vi "HysteresisExample.vi"() -> ()   [LabVIEW 2020]
panel:
  out "Output":dbl
  out "Waveform Chart":dbl(graph)
  out "ON":bool
  in  "High threshold":dbl=11.0
  in  "Low threshold":dbl=9.0
  in  "Start":bool
  in  "stop":bool
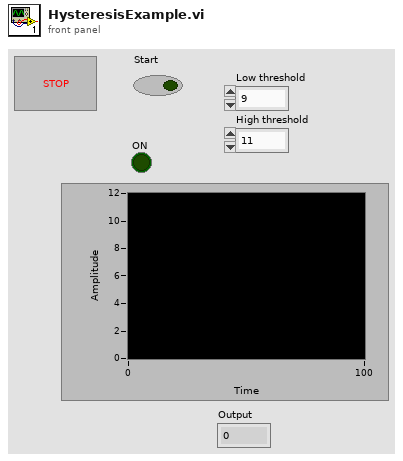
[diagram p1: front panel]
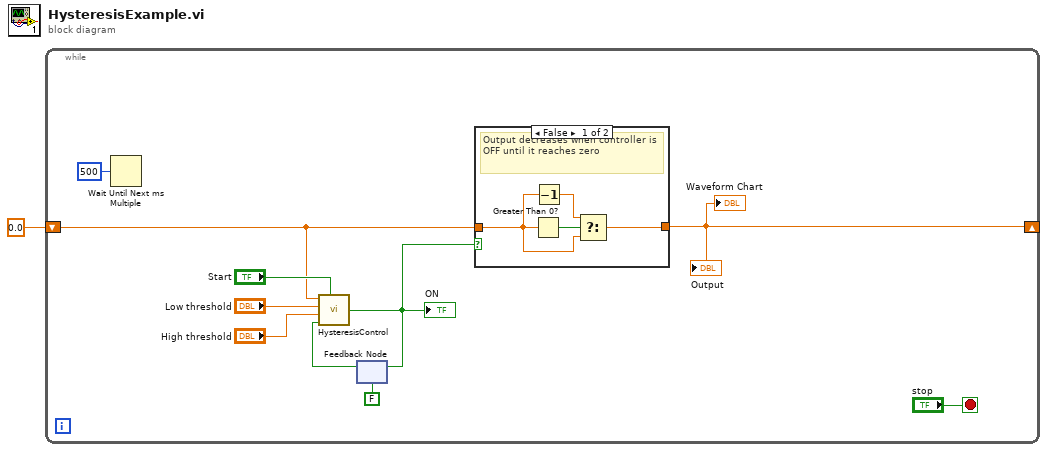
[diagram p0: block diagram]
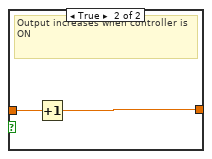
[diagram p2: hidden frame]
diagram:
  n1 = while {
    shift-right: [w6] -> _
    shift-left: 0.0 -> [w5]
    stop <- "stop" stop-if-true
    n2 = Wait Until Next ms Multiple(millisecond multiple=u32 500) -> ()  [unwired: 1 out]
    n3 = feedback #1(FALSE ("Run out")) -> (w3:bool)
    n4 = call "HysteresisControl.vi"("Process variable"=w5, "Low threshold"="Low threshold", "High threshold"="High threshold", "Run in"=w3, "Start"="Start") -> ("Run out"=w4:bool)
    "ON" <- w4
    n5 = feedback-in #1(w4) -> ()
    n6 = case shown="False" w4 {
      tunnel: w5 -> [w13 w17]
      tunnel: [w12 w16] -> w6
      frame False {
        # "Output decreases when controller is OFF until it reaches zero"
        n7 = Greater Than 0?(x=w13) -> (x > 0?=w15:bool)
        n8 = Decrement(x=w13) -> (x-1=w14:dbl)
        n9 = Select(t=w14, s=w15, f=w13) -> (s? t:f=w12:dbl)
      }
      frame True {
        # "Output increases when controller is ON"
        n10 = Increment(x=w17) -> (x+1=w16:dbl)
      }
    }
    "Waveform Chart" <- w6
    "Output" <- w6
  }
